vi "dash safety data FG.vi"(2 "Mechanism":enum16{"Arm", "Drive Train"}(ring), 3 "Drive Safety Data":T1, 4 "Arm Safety Data":T2, 5 "Menu":T3) -> (0 "Drive Safety Data Out":T1, 1 "Arm Safety Data Out":T2)   [LabVIEW 2013]
uses:
  typedefs/fg_typedef.ctl
  typedefs/Dashboard/dashboard safety status data.ctl
  typedefs/Dashboard/drive safety.ctl
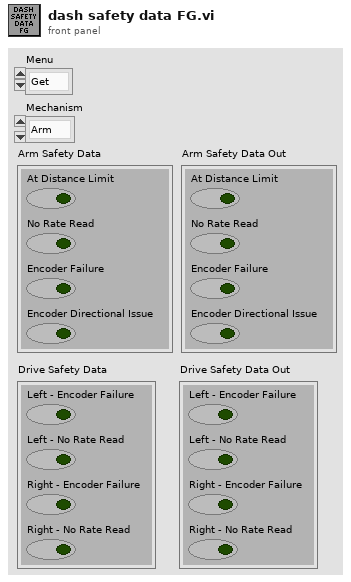
[diagram p1: front panel]
types:
  T1 = typedef "drive safety.ctl" = cluster{"Left - Encoder Failure":bool, "Left - No Rate Read":bool, "Right - Encoder Failure":bool, "Right - No Rate Read":bool}
  T2 = typedef "dashboard safety status data.ctl" = cluster{"At Distance Limit":bool, "No Rate Read":bool, "Encoder Failure":bool, "Encoder Directional Issue":bool}
  T3 = typedef "fg_typedef.ctl" = enum16{"Get", "Set"}
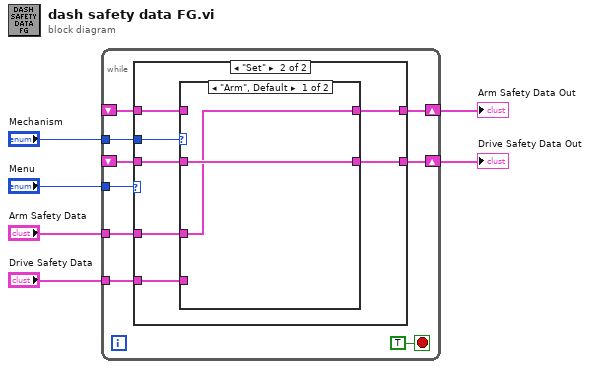
[diagram p0: block diagram]
diagram:
  n1 = while {
    tunnel: "Menu" -> [w14]
    shift-right: [w11] -> w4
    shift-left: _ -> [w13]
    tunnel: "Arm Safety Data" -> [w12]
    shift-right: [w8] -> w1
    shift-left: _ -> [w7]
    tunnel: "Mechanism" -> [w10]
    tunnel: "Drive Safety Data" -> [w9]
    stop <- TRUE stop-if-true
    n2 = case shown="\"Set\"" w14 {
      tunnel: w13 -> [w17 w19]
      tunnel: [w17 w21] -> w11
      tunnel: w12 -> [_ w23]
      tunnel: w10 -> [_ w24]
      tunnel: w9 -> [_ w22]
      tunnel: [w16 w20] -> w8
      tunnel: w7 -> [w16 w18]
      frame "Get", Default {
      }
      frame "Set" {
        n3 = case shown="\"Arm\", Default" w24 {
          tunnel: w23 -> [w25 _]
          tunnel: w22 -> [_ w28]
          tunnel: [w25 w27] -> w21
          tunnel: [w26 w28] -> w20
          tunnel: w19 -> [_ w27]
          tunnel: w18 -> [w26 _]
          frame "Arm", Default {
          }
          frame "Drive Train" {
          }
        }
      }
    }
  }
  "Arm Safety Data Out" <- w4
  "Drive Safety Data Out" <- w1
